vi "DecodeSOSPackage.vi"(8 "error in":errorcluster, 10 "Array":u8[](array[numeric]) format="%02x") -> (0 "error IO":errorcluster, 2 "Vector Flags":cluster{"id":dbl, "flag":bool}[](array[cluster]))   [LabVIEW 2017]
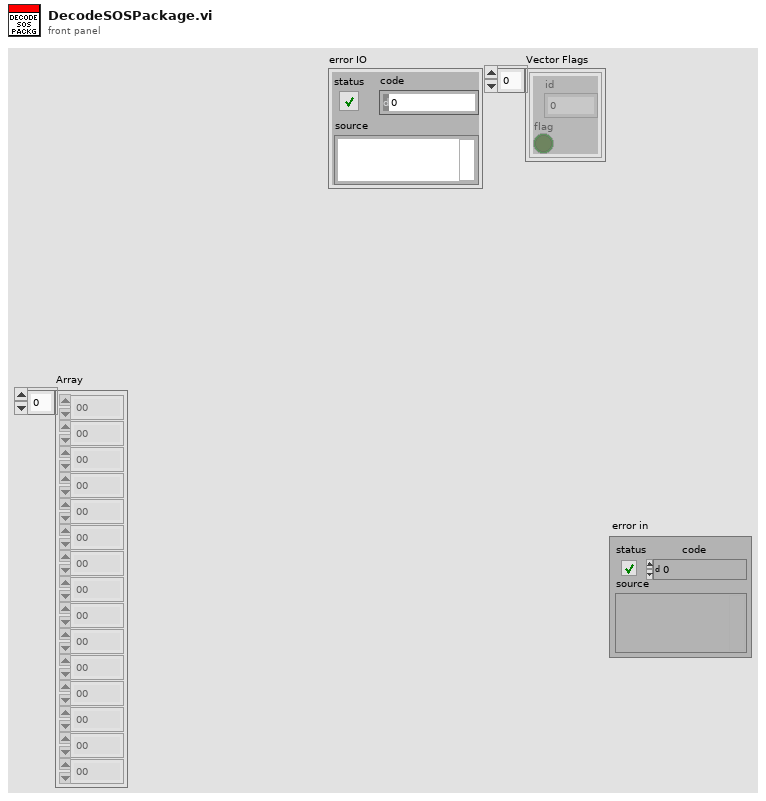
[diagram p1: front panel]
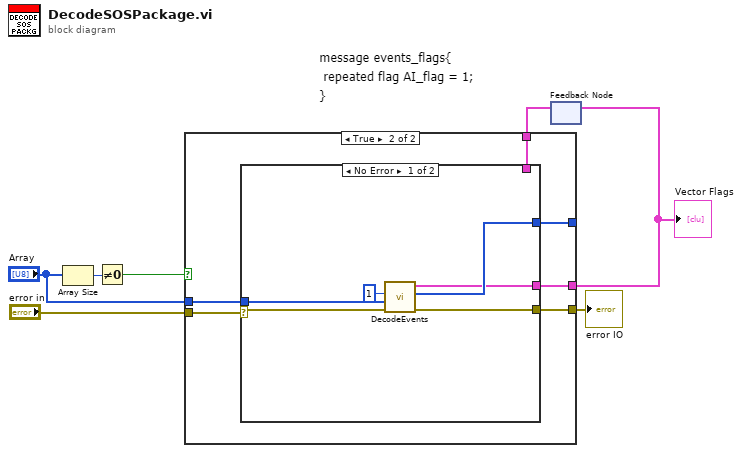
[diagram p0: block diagram]
diagram:
  n1 = Array Size(array="Array") -> (size(s)=w7:i32)
  n2 = Not Equal To 0?(x=w7) -> (x != 0?=w6:bool)
  n3 = feedback #1() -> (w1:cluster{"id":dbl, "flag":bool}[])  [unwired: 1 in]
  n4 = case shown="True" w6 {
    tunnel: "error in" -> [w10 w16]
    tunnel: "Array" -> [w9 w15]
    tunnel: [w10 w14] -> w3
    tunnel: [w9 w13] -> _
    tunnel: [w8 w12] -> w2
    tunnel: w1 -> [w8 w11]
    frame False {
    }
    frame True {
      n5 = case shown="No Error" w16 {
        selector: w16 -> [w20 w25]
        tunnel: w15 -> [w22 w24]
        tunnel: [w19 w25] -> w14
        tunnel: [w18 w24] -> w13
        tunnel: [w17 w23] -> w12
        tunnel: w11 -> [_ w23]
        frame No Error {
          n6 = call "DecodeEvents.vi"("error in"=w20, "array"=w22, "Key"=1) -> ("error out"=w19:errorcluster, "array w/ subset deleted out"=w18:u8[], "Vector Flags"=w17:cluster{"id":dbl, "flag":bool}[])  [unwired: 6 in]
        }
        frame Error {
        }
      }
    }
  }
  "error IO" <- w3
  "Vector Flags" <- w2
  n7 = feedback-in #1(w2) -> ()
